vi "XYZ calculator.vi"(5 "X(g)":dbl, 7 "Y(g)":dbl, 9 "Z(g)":dbl) -> (4 "Magnitude XY(g)":dbl, 6 "Angle x-xy":dbl, 8 "Magnitude XYZ(g)":dbl, 10 "Angle z-xyz":dbl, 15 "Angle x - xy w sign":dbl)   [LabVIEW 2011]
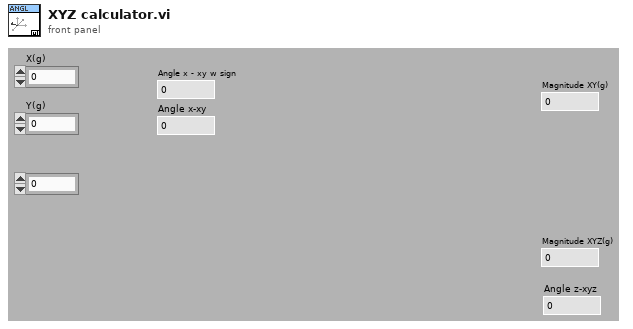
[diagram p1: front panel]
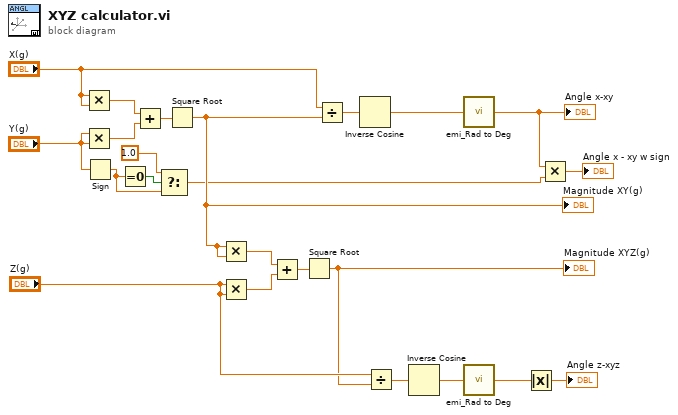
[diagram p0: block diagram]
diagram:
  n1 = Multiply(x="X(g)", y="X(g)") -> (x*y=w23:dbl)
  n2 = Multiply(x="Y(g)", y="Y(g)") -> (x*y=w22:dbl)
  n3 = Sign(1:"Y(g)") -> (0:w5:dbl)
  n4 = Equal To 0?(x=w5) -> (x = 0?=w6:bool)
  n5 = Add(x=w23, y=w22) -> (x+y=w21:dbl)
  n6 = Select(t=1.0, s=w6, f=w5) -> (s? t:f=w2:dbl)
  n7 = Square Root(x=w21) -> (sqrt(x)=w15:dbl)
  "Magnitude XY(g)" <- w15
  n8 = Multiply(x=w15, y=w15) -> (x*y=w16:dbl)
  n9 = Multiply(x="Z(g)", y="Z(g)") -> (x*y=w17:dbl)
  n10 = Add(x=w16, y=w17) -> (x+y=w18:dbl)
  n11 = Square Root(x=w18) -> (sqrt(x)=w12:dbl)
  "Magnitude XYZ(g)" <- w12
  n12 = Divide(x="X(g)", y=w15) -> (x/y=w19:dbl)
  n13 = Inverse Cosine(1:w19) -> (0:w8:dbl)
  n14 = Divide(x="Z(g)", y=w12) -> (x/y=w14:dbl)
  n15 = Inverse Cosine(1:w14) -> (0:w10:dbl)
  n16 = call "emi_Rad to Deg.vi"("Rad"=w8) -> ("Deg"=w3:dbl)  [unwired: 14 in]
  "Angle x-xy" <- w3
  n17 = call "emi_Rad to Deg.vi"("Rad"=w10) -> ("Deg"=w9:dbl)  [unwired: 14 in]
  n18 = Absolute Value(x=w9) -> (abs(x)=→"Angle z-xyz":dbl)
  n19 = Multiply(x=w3, y=w2) -> (x*y=→"Angle x - xy w sign":dbl)
